vi "Move stages visa control.vi"() -> ()   [LabVIEW 2020]
uses:
  <vilib>/Instr/_visa.llb/VISA Configure Serial Port (Instr).vi
panel:
  in  "stop":bool
  out "Last time reading":u32=1502
  out "BG Task":bool
  in  "Step speed":i32(ring)=3 items=["Off", "Slow", "Medium", "Fast"]
  in  "Direction":bool
  out "In Motion":bool
  in  "Limit travel time":bool
  in  "Travel time (sec)":dbl=11.0
  in  "Reset timer":bool
  out "Elapsed time (msec)":u32
  in  "Go/Stop":bool
  in  "Stage Address":i32(ring)=3 items=["Ground Electrode Stage"=4, "Horizontal Stage"=3, "Vertical Stage"=2, "Electrode Stage"=1]
  out "error out":errorcluster
  out "Last time":u32=1204713779
  # "Horizontal"
  # "Down"
  # "In"
  # "Out"
  # "In"
  # "Out"
  # "Up"
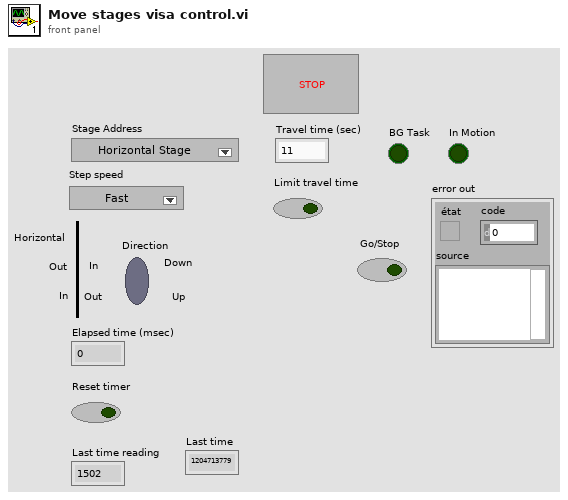
[diagram p1: front panel]
types:
  T1 = enum8{"Enabled", "Disabled", "Disabled and Grayed Out"}
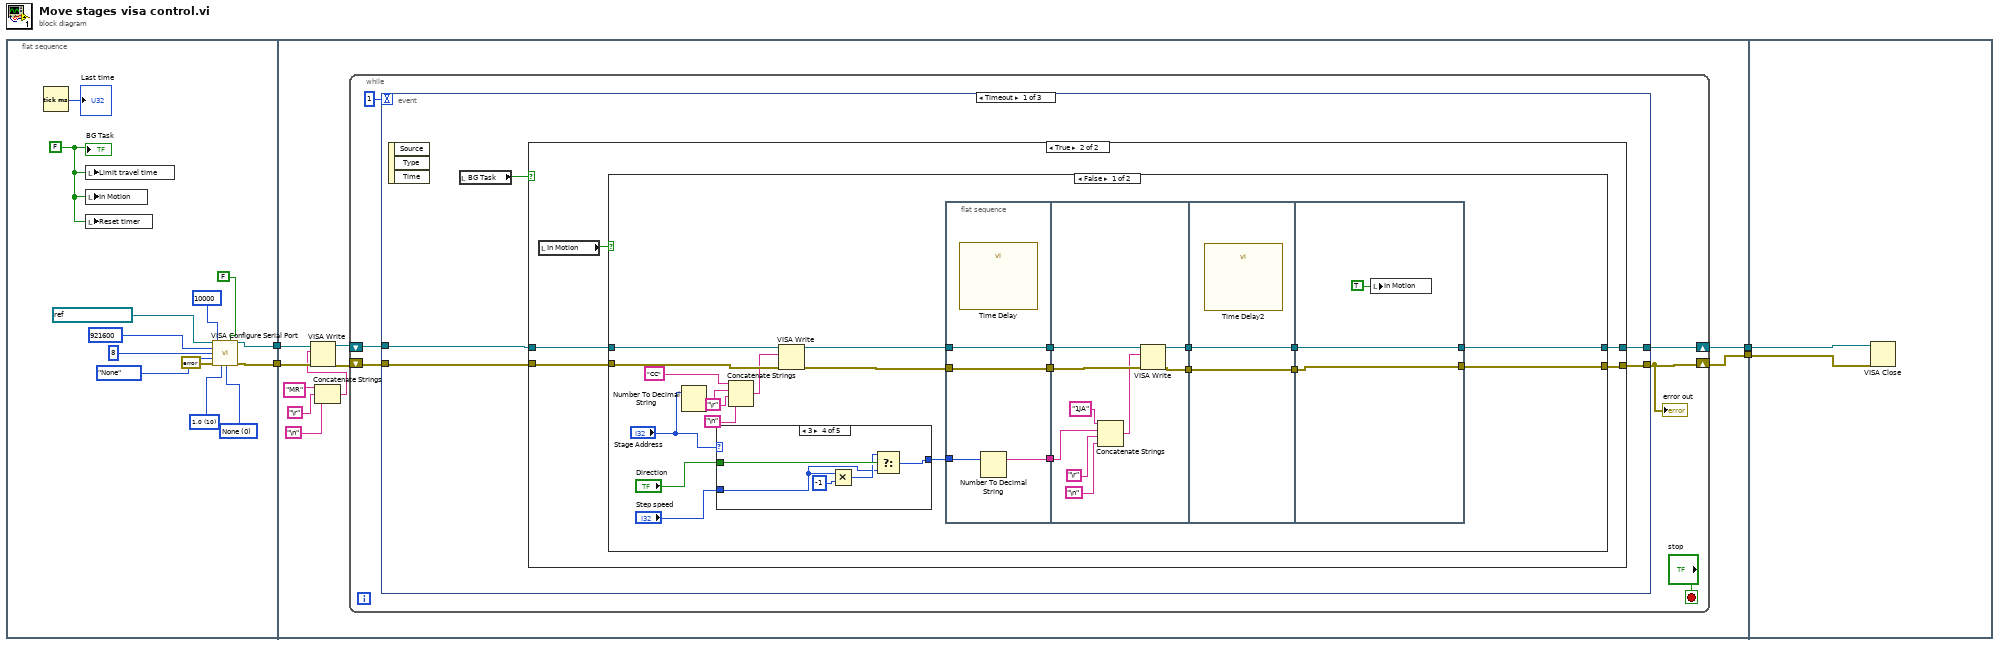
[diagram p0: block diagram]
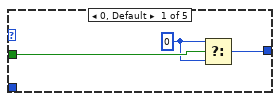
[diagram p3: hidden frame]
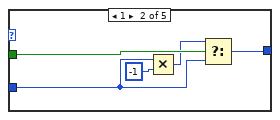
[diagram p4: hidden frame]
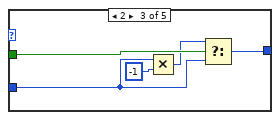
[diagram p5: hidden frame]
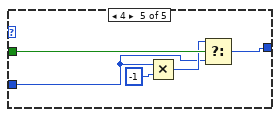
[diagram p6: hidden frame]
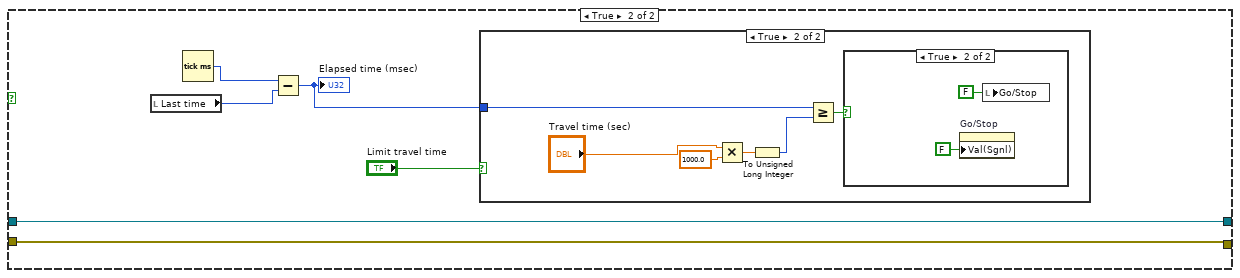
[diagram p7: hidden frame]
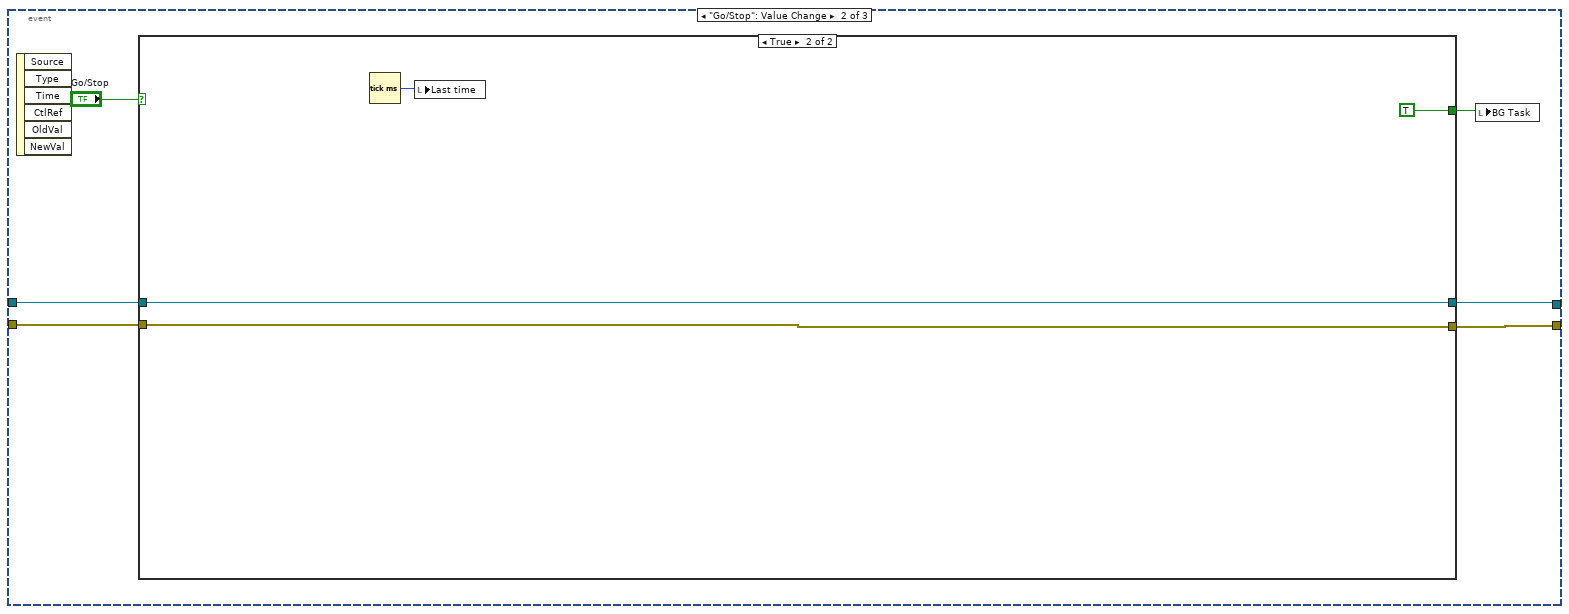
[diagram p10: hidden frame]
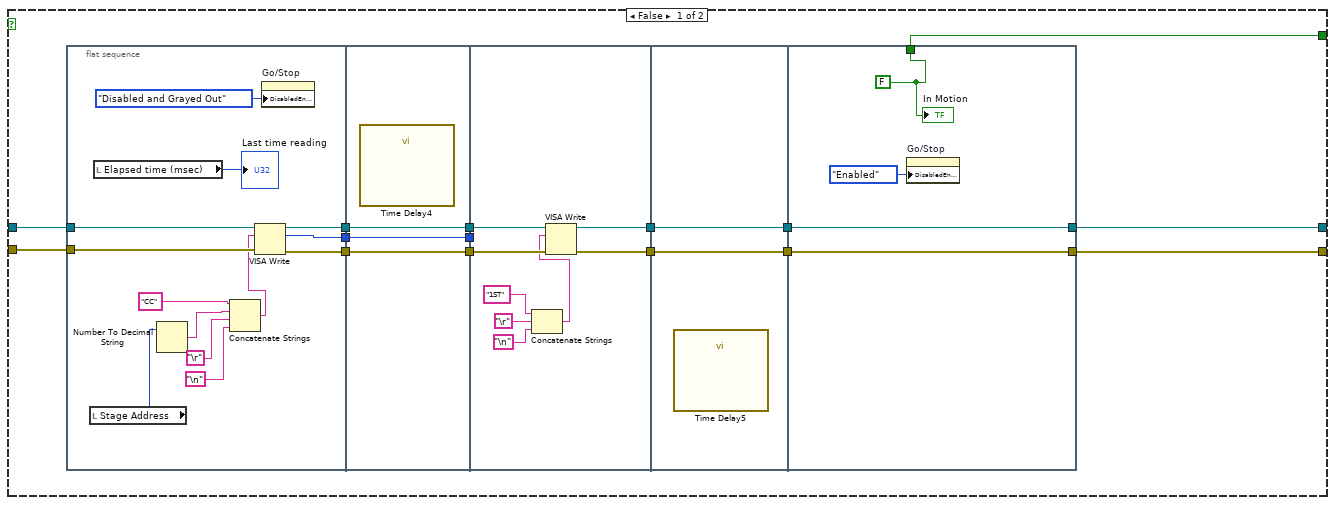
[diagram p11: hidden frame]
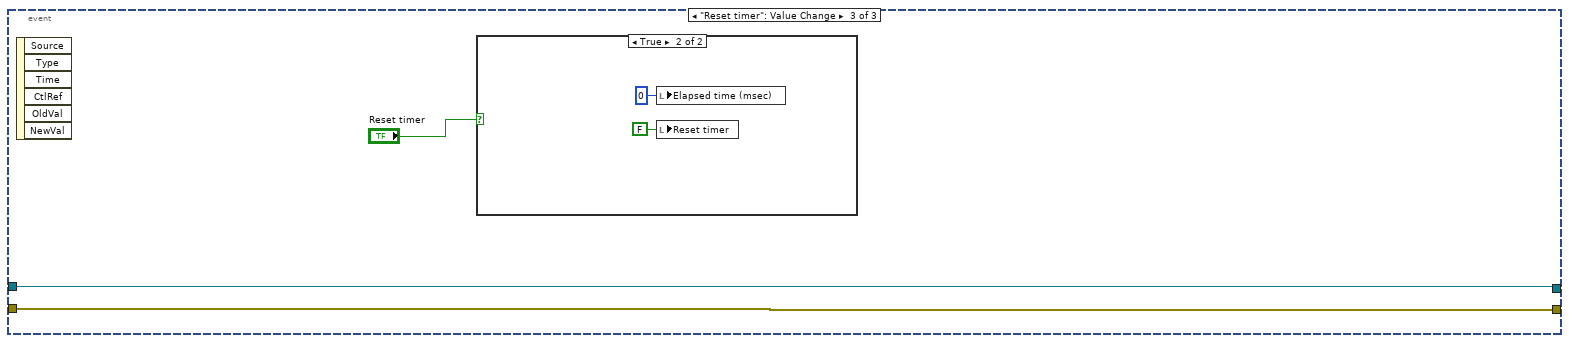
[diagram p12: hidden frame]
diagram:
  n1 = flat-sequence {
    tunnel: [w15] -> w4
    tunnel: [w14] -> w3
    tunnel: w4 -> [w25]
    tunnel: w3 -> [w24]
    tunnel: [w27] -> w2
    tunnel: [w26] -> w1
    tunnel: w2 -> [w183]
    tunnel: w1 -> [w184]
    frame #0 {
      w6 = u16 0 items=["None", "XON/XOFF", "RTS/CTS", "XON/XOFF & RTS/CTS", "DTR/DSR", "XON/XOFF & DTR/DSR"] ("flow control (0:none)")
      w7 = u16 10 items=["1.0"=10, "1.5"=15, "2.0"=20] ("stop bits (10: 1 bit)")
      w16 = FALSE
      n2 = Tick Count (ms)() -> (millisecond timer value=→"Last time":u32)
      n3 = local write "Limit travel time"(w16) -> ()
      n4 = local write "In Motion"(w16) -> ()
      n5 = local write "Reset timer"(w16) -> ()
      n6 = call-poly "VISA Configure Serial Port"("VISA resource name"=refnum<visa-resource-name> "ASRL3::INSTR", "timeout (10sec)"=u32 10000, "Enable Termination\nChar (T)"=FALSE ("Enable Termination\nChar (T)"), "baud rate (9600)"=u32 921600, "data bits (8)"=u16 8, "parity (0:none)"=enum16{"None", "Odd", "Even", "Mark", "Space"}."None", "error in (no error)"=errorcluster {"status"=FALSE, "code"=0, "source"=""}, "stop bits (10: 1 bit)"=w7, "flow control (0:none)"=w6) -> ("VISA resource name out"=w15:refnum<visa-resource-name>, "error out"=w14:errorcluster)  [unwired: 5 in]
      "BG Task" <- w16
    }
    frame #1 {
      n7 = Concatenate Strings("MR" ("write buffer"), "\r", "\n") -> (w18:string)
      n8 = VISA Write(VISA resource name=w25, write buffer=w18, error in (no error)=w24) -> (VISA resource name out=w23:refnum<visa-resource-name>, error out=w22:errorcluster)  [unwired: 1 out]
      n9 = while {
        shift-right: [w30] -> w26
        shift-left: w23 -> [w32]
        shift-right: [w29] -> w27
        shift-left: w22 -> [w31]
        stop <- "stop" stop-if-true
        n10 = event shown="[0] Timeout" {
          selector: _ -> [_ _ _]
          dyn-events: _ -> [_ _ _]
          timeout: 1 -> [_ _ _]
          tunnel: w32 -> [w35 w127 w179]
          tunnel: w31 -> [w34 w126 w178]
          tunnel: [w38 w124 w178] -> w29
          tunnel: [w37 w125 w179] -> w30
          event Timeout {
            n11 = event-data() -> ()  [unwired: 1 in, 3 out]
            n12 = local read "BG Task"() -> (w36:bool)
            n13 = case shown="True" w36 {
              tunnel: [w39 w41] -> w38
              tunnel: [w40 w45] -> w37
              tunnel: w35 -> [w40 w44]
              tunnel: w34 -> [w39 w42]
              frame False {
              }
              frame True {
                n14 = local read "In Motion"() -> (w43:bool)
                n15 = case shown="False" w43 {
                  tunnel: [w49 w114] -> w45
                  tunnel: w44 -> [w67 w114]
                  tunnel: [w48 w109] -> w41
                  tunnel: w42 -> [w58 w109]
                  frame False {
                    n16 = Number To Decimal String(number="Stage Address") -> (decimal integer string=w55:string)  [unwired: 1 in]
                    n17 = case shown="3" "Stage Address" {
                      tunnel: "Step speed" -> [_ w90 w94 w99 w104]
                      tunnel: [w87 w92 w96 w101 w106] -> w59
                      tunnel: "Direction" -> [w88 w91 w97 w102 w107]
                      frame 0, Default {
                        w86 = 0 ("y")
                        n18 = Select(t=w86, s=w88, f=w86) -> (s? t:f=w87:i32)
                      }
                      frame 1 {
                        n19 = Multiply(x=w90, y=-1) -> (x*y=w89:i32)
                        n20 = Select(t=w89, s=w91, f=w90) -> (s? t:f=w92:i32)
                      }
                      frame 2 {
                        n21 = Multiply(x=w94, y=-1) -> (x*y=w95:i32)
                        n22 = Select(t=w95, s=w97, f=w94) -> (s? t:f=w96:i32)
                      }
                      frame 3 {
                        n23 = Multiply(x=w99, y=-1) -> (x*y=w100:i32)
                        n24 = Select(t=w100, s=w102, f=w99) -> (s? t:f=w101:i32)
                      }
                      frame 4 {
                        n25 = Multiply(x=w104, y=-1) -> (x*y=w105:i32)
                        n26 = Select(t=w105, s=w107, f=w104) -> (s? t:f=w106:i32)
                      }
                    }
                    n27 = Concatenate Strings("CC", w55, "\r", "\n") -> (w52:string)
                    n28 = VISA Write(VISA resource name=w67, write buffer=w52, error in (no error)=w58) -> (VISA resource name out=w63:refnum<visa-resource-name>, error out=w56:errorcluster)  [unwired: 1 out]
                    n29 = flat-sequence {
                      tunnel: [w71] -> w64
                      tunnel: w63 -> [w71]
                      tunnel: [w68] -> w60
                      tunnel: w59 -> [w70]
                      tunnel: [w69] -> w57
                      tunnel: w56 -> [w69]
                      tunnel: w64 -> [w80]
                      tunnel: [w79] -> w61
                      tunnel: w60 -> [w77]
                      tunnel: w57 -> [w78]
                      tunnel: [w74] -> w50
                      tunnel: [w82] -> w62
                      tunnel: w61 -> [w82]
                      tunnel: [w81] -> w51
                      tunnel: w50 -> [w81]
                      tunnel: w62 -> [w84]
                      tunnel: w51 -> [w83]
                      tunnel: [w84] -> w49
                      tunnel: [w83] -> w48
                      frame #0 {
                        n30 = call "Time Delay"() -> ()  [unwired: 11 in, 1 out]
                        n31 = Number To Decimal String(number=w70) -> (decimal integer string=w68:string)  [unwired: 1 in]
                      }
                      frame #1 {
                        n32 = Concatenate Strings("1JA", w77, "\r", "\n") -> (w75:string)
                        n33 = VISA Write(VISA resource name=w80, write buffer=w75, error in (no error)=w78) -> (VISA resource name out=w79:refnum<visa-resource-name>, error out=w74:errorcluster)  [unwired: 1 out]
                      }
                      frame #2 {
                        n34 = call "Time Delay2"() -> ()  [unwired: 11 in, 1 out]
                      }
                      frame #3 {
                        n35 = local write "In Motion"(TRUE ("In Motion")) -> ()
                      }
                    }
                  }
                  frame True {
                    n36 = local read "Last time"() -> (w112:u32)
                    n37 = Tick Count (ms)() -> (millisecond timer value=w113:u32)
                    n38 = Subtract(x=w113, y=w112) -> (x-y=w110:u32)
                    "Elapsed time (msec)" <- w110
                    n39 = case shown="True" "Limit travel time" {
                      tunnel: w110 -> [_ w117]
                      frame False {
                      }
                      frame True {
                        n40 = Multiply(x="Travel time (sec)", y=1000.0) -> (x*y=w120:dbl)
                        n41 = To Unsigned Long Integer(number=w120) -> (unsigned 32bit integer=w118:u32)
                        n42 = Greater Or Equal?(x=w117, y=w118) -> (x >= y?=w116:bool)
                        n43 = case shown="True" w116 {
                          frame False {
                          }
                          frame True {
                            n44 = property on="Go/Stop" class="Bool (strict)"("Val(Sgnl)"=FALSE ("Value (Signaling)")) -> ()  [unwired: 2 in, 2 out]
                            n45 = local write "Go/Stop"(FALSE ("Go/Stop")) -> ()
                          }
                        }
                      }
                    }
                  }
                }
              }
            }
          }
          event "Go/Stop": Value Change {
            n46 = event-data() -> ()  [unwired: 1 in, 6 out]
            n47 = case shown="True" "Go/Stop" {
              tunnel: w127 -> [w143 w176]
              tunnel: w126 -> [w142 w175]
              tunnel: [w136 w176] -> w125
              tunnel: [w131 w175] -> w124
              tunnel: [w135 TRUE] -> w123
              frame False {
                n48 = flat-sequence {
                  tunnel: w143 -> [w156]
                  tunnel: w142 -> [w151]
                  tunnel: [w153] -> w140
                  tunnel: [w152] -> w138
                  tunnel: [w150] -> w133
                  tunnel: [w159] -> w141
                  tunnel: w140 -> [w159]
                  tunnel: [w158] -> w139
                  tunnel: w138 -> [w158]
                  tunnel: [w157] -> w134
                  tunnel: w133 -> [w157]
                  tunnel: w141 -> [w167]
                  tunnel: w139 -> [_]
                  tunnel: [w166] -> w137
                  tunnel: w134 -> [w165]
                  tunnel: [w164] -> w132
                  tunnel: w137 -> [w169]
                  tunnel: w132 -> [w168]
                  tunnel: [w169] -> w130
                  tunnel: [w168] -> w129
                  tunnel: [w171] -> w136
                  tunnel: [w172] -> w135
                  tunnel: [w170] -> w131
                  tunnel: w130 -> [w171]
                  tunnel: w129 -> [w170]
                  frame #0 {
                    n49 = local read "Stage Address"() -> (w149:i32)
                    n50 = local read "Elapsed time (msec)"() -> (→"Last time reading":u32)
                    n51 = Number To Decimal String(number=w149) -> (decimal integer string=w148:string)  [unwired: 1 in]
                    n52 = Concatenate Strings("CC", w148, "\r", "\n") -> (w146:string)
                    n53 = VISA Write(VISA resource name=w156, write buffer=w146, error in (no error)=w151) -> (VISA resource name out=w153:refnum<visa-resource-name>, return count=w152:u32, error out=w150:errorcluster)
                    n54 = property on="Go/Stop" class="Bool (strict)"("DisabledEnum"=T1."Disabled and Grayed Out" ("Disabled")) -> ()  [unwired: 2 in, 2 out]
                  }
                  frame #1 {
                    n55 = call "Time Delay4"() -> ()  [unwired: 11 in, 1 out]
                  }
                  frame #2 {
                    n56 = Concatenate Strings("1ST", "\r", "\n") -> (w160:string)
                    n57 = VISA Write(VISA resource name=w167, write buffer=w160, error in (no error)=w165) -> (VISA resource name out=w166:refnum<visa-resource-name>, error out=w164:errorcluster)  [unwired: 1 out]
                  }
                  frame #3 {
                    n58 = call "Time Delay5"() -> ()  [unwired: 11 in, 1 out]
                  }
                  frame #4 {
                    w172 = FALSE
                    n59 = property on="Go/Stop" class="Bool (strict)"("DisabledEnum"=T1."Enabled" ("Disabled")) -> ()  [unwired: 2 in, 2 out]
                    "In Motion" <- w172
                  }
                }
              }
              frame True {
                n60 = Tick Count (ms)() -> (millisecond timer value=w177:u32)
                n61 = local write "Last time"(w177) -> ()
              }
            }
            n62 = local write "BG Task"(w123) -> ()
          }
          event "Reset timer": Value Change {
            n63 = event-data() -> ()  [unwired: 1 in, 6 out]
            n64 = case shown="True" "Reset timer" {
              frame False {
              }
              frame True {
                n65 = local write "Elapsed time (msec)"(u32 0 ("Elapsed time (msec)")) -> ()
                n66 = local write "Reset timer"(FALSE ("Reset timer")) -> ()
              }
            }
          }
        }
        "error out" <- w29
      }
    }
    frame #2 {
      n67 = VISA Close(VISA resource name=w184, error in (no error)=w183) -> ()  [unwired: 1 out]
    }
  }
